vi "NUMPAD1_9(ПРОГРАММА).vi"(6 "МИНИМАЛЬНОЕ ЗНАЧЕНИЕ":dbl, 7 "МАКСИМАЛЬНОЕ ЗНАЧЕНИЕ":dbl, 8 "ДЛИННА СЛОВА":i8, 11 "ТЕКУЩЕЕ ЗНАЧЕНИЕ":string) -> (2 "НОВОЕ ЗНАЧЕНИЕ":string)   [LabVIEW 2016, in "Library.lvlib"]
uses:
  Granule-2000AT/PC/Library.lvlib
panel:
  in  ",":bool
  in  "ТЕМП":string
  in  "ОТМЕНА":bool
  in  "ВВОД":bool
  in  "УДАЛИТЬ":bool
  in  "0":bool
  in  "9":bool
  in  "8":bool
  in  "7":bool
  in  "6":bool
  in  "5":bool
  in  "4":bool
  in  "3":bool
  in  "2":bool
  in  "1":bool
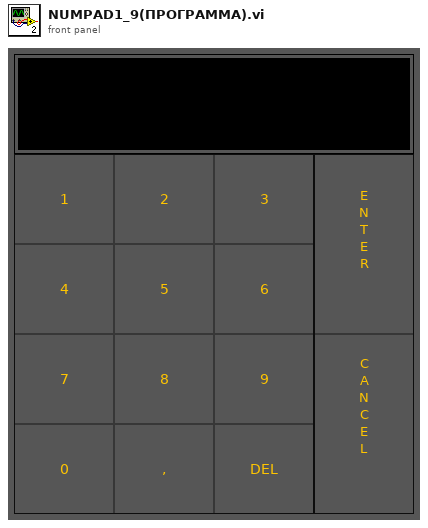
[diagram p1: front panel]
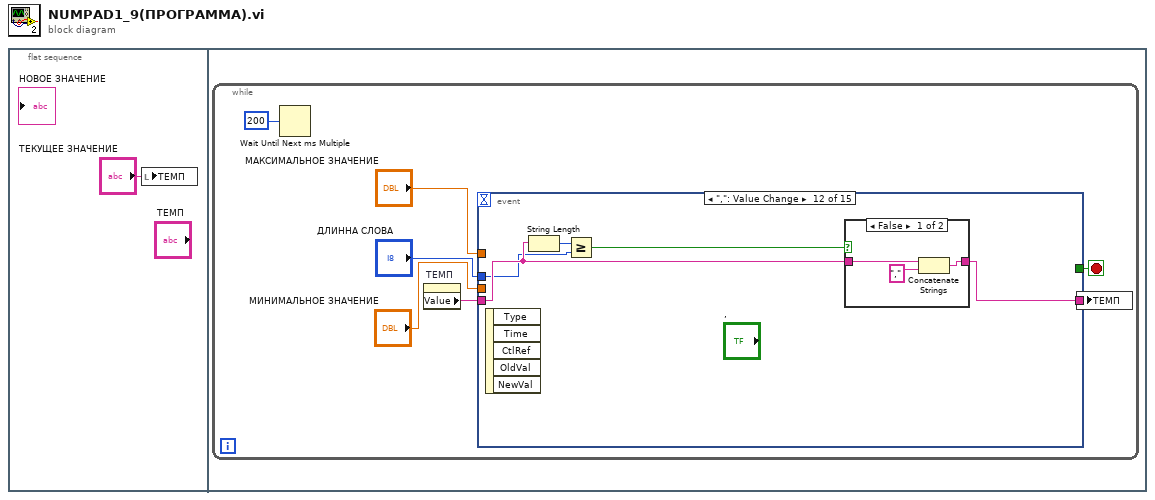
[diagram p0: block diagram]
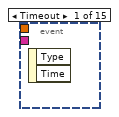
[diagram p2: hidden frame]
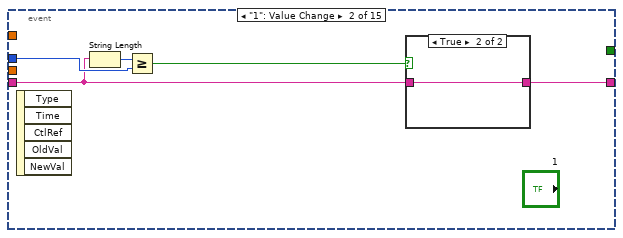
[diagram p3: hidden frame]
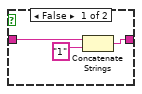
[diagram p4: hidden frame]
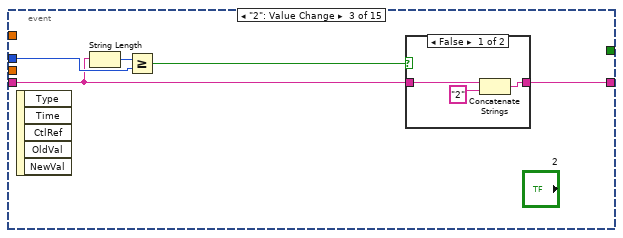
[diagram p5: hidden frame]
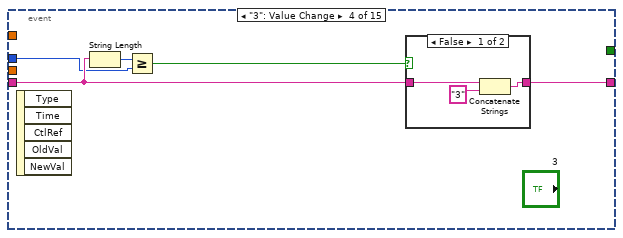
[diagram p7: hidden frame]
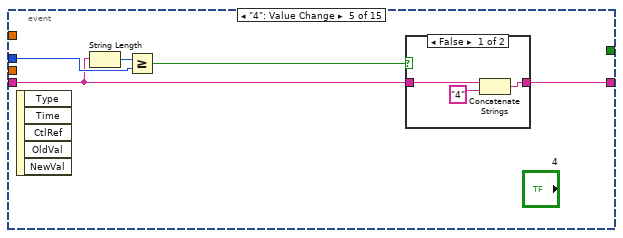
[diagram p9: hidden frame]
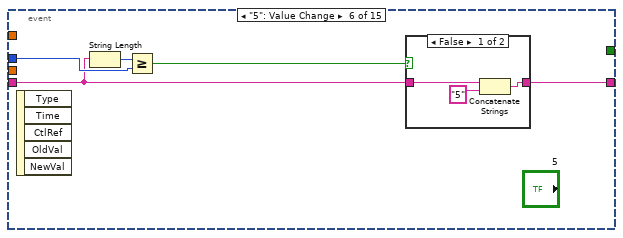
[diagram p11: hidden frame]
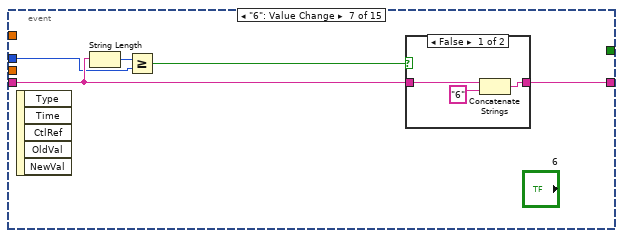
[diagram p13: hidden frame]
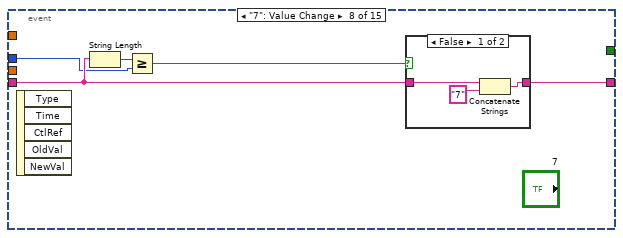
[diagram p15: hidden frame]
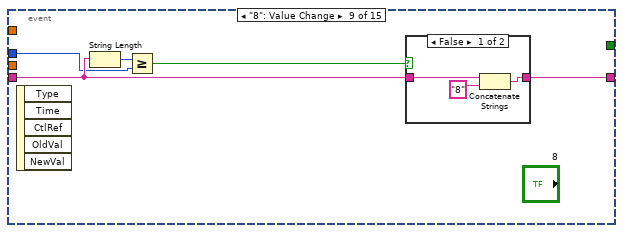
[diagram p17: hidden frame]
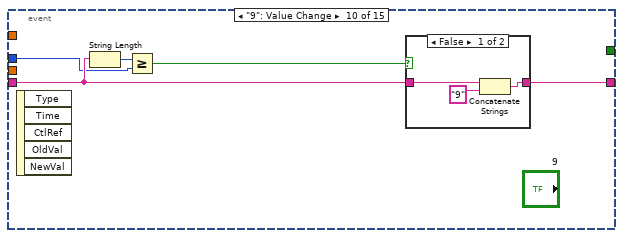
[diagram p19: hidden frame]
diagram:
  n1 = flat-sequence {
    frame #0 {
      n2 = local write "ТЕМП"("ТЕКУЩЕЕ ЗНАЧЕНИЕ") -> ()
    }
    frame #1 {
      n3 = while {
        stop <- w3 stop-if-true
        n4 = Wait Until Next ms Multiple(millisecond multiple=u32 200) -> ()  [unwired: 1 out]
        n5 = property on="ТЕМП" class="Str"() -> ("Value"=w7:string)  [unwired: 2 in, 2 out]
        n6 = event shown="[11] \",\": Value Change" {
          selector: _ -> [_ _ _ _ _ _ _ _ _ _ _ _ _ _ _]
          dyn-events: _ -> [_ _ _ _ _ _ _ _ _ _ _ _ _ _ _]
          timeout: _ -> [_ _ _ _ _ _ _ _ _ _ _ _ _ _ _]
          tunnel: "ДЛИННА СЛОВА" -> [_ w12 w20 w28 w38 w47 w55 w64 w72 w81 w91 w100 _ _ _]
          tunnel: w7 -> [_ w10 w19 w29 w37 w45 w56 w65 w74 w83 w92 w101 w109 w114 _]
          tunnel: [_ w9 w18 w27 w36 w46 w54 w63 w73 w82 w90 w99 w108 w112 _] -> w6
          tunnel: "МАКСИМАЛЬНОЕ ЗНАЧЕНИЕ" -> [_ _ _ _ _ _ _ _ _ _ _ _ _ w117 _]
          tunnel: "МИНИМАЛЬНОЕ ЗНАЧЕНИЕ" -> [_ _ _ _ _ _ _ _ _ _ _ _ _ w116 _]
          tunnel: [_ _ _ _ _ _ _ _ _ _ _ _ _ w113 "ОТМЕНА"] -> w3
          event Timeout {
            n7 = event-data() -> ()  [unwired: 1 in, 2 out]
          }
          event "1": Value Change {
            n8 = event-data() -> ()  [unwired: 1 in, 5 out]
            n9 = String Length(string=w10) -> (length=w13:i32)
            n10 = Greater Or Equal?(x=w13, y=w12) -> (x >= y?=w11:bool)
            n11 = case shown="True" w11 {
              tunnel: w10 -> [w16 w17]
              tunnel: [w14 w17] -> w9
              frame False {
                n12 = Concatenate Strings(w16, "1" ("string")) -> (w14:string)
              }
              frame True {
              }
            }
          }
          event "2": Value Change {
            n13 = event-data() -> ()  [unwired: 1 in, 5 out]
            n14 = String Length(string=w19) -> (length=w22:i32)
            n15 = Greater Or Equal?(x=w22, y=w20) -> (x >= y?=w21:bool)
            n16 = case shown="False" w21 {
              tunnel: w19 -> [w25 w26]
              tunnel: [w23 w26] -> w18
              frame False {
                n17 = Concatenate Strings(w25, "2" ("string")) -> (w23:string)
              }
              frame True {
              }
            }
          }
          event "3": Value Change {
            n18 = event-data() -> ()  [unwired: 1 in, 5 out]
            n19 = String Length(string=w29) -> (length=w31:i32)
            n20 = Greater Or Equal?(x=w31, y=w28) -> (x >= y?=w30:bool)
            n21 = case shown="False" w30 {
              tunnel: w29 -> [w34 w35]
              tunnel: [w32 w35] -> w27
              frame False {
                n22 = Concatenate Strings(w34, "3" ("string")) -> (w32:string)
              }
              frame True {
              }
            }
          }
          event "4": Value Change {
            n23 = event-data() -> ()  [unwired: 1 in, 5 out]
            n24 = String Length(string=w37) -> (length=w40:i32)
            n25 = Greater Or Equal?(x=w40, y=w38) -> (x >= y?=w39:bool)
            n26 = case shown="False" w39 {
              tunnel: w37 -> [w43 w44]
              tunnel: [w41 w44] -> w36
              frame False {
                n27 = Concatenate Strings(w43, "4" ("string")) -> (w41:string)
              }
              frame True {
              }
            }
          }
          event "5": Value Change {
            n28 = event-data() -> ()  [unwired: 1 in, 5 out]
            n29 = String Length(string=w45) -> (length=w49:i32)
            n30 = Greater Or Equal?(x=w49, y=w47) -> (x >= y?=w48:bool)
            n31 = case shown="False" w48 {
              tunnel: w45 -> [w52 w53]
              tunnel: [w50 w53] -> w46
              frame False {
                n32 = Concatenate Strings(w52, "5" ("string")) -> (w50:string)
              }
              frame True {
              }
            }
          }
          event "6": Value Change {
            n33 = event-data() -> ()  [unwired: 1 in, 5 out]
            n34 = String Length(string=w56) -> (length=w58:i32)
            n35 = Greater Or Equal?(x=w58, y=w55) -> (x >= y?=w57:bool)
            n36 = case shown="False" w57 {
              tunnel: w56 -> [w61 w62]
              tunnel: [w59 w62] -> w54
              frame False {
                n37 = Concatenate Strings(w61, "6" ("string")) -> (w59:string)
              }
              frame True {
              }
            }
          }
          event "7": Value Change {
            n38 = event-data() -> ()  [unwired: 1 in, 5 out]
            n39 = String Length(string=w65) -> (length=w67:i32)
            n40 = Greater Or Equal?(x=w67, y=w64) -> (x >= y?=w66:bool)
            n41 = case shown="False" w66 {
              tunnel: w65 -> [w70 w71]
              tunnel: [w68 w71] -> w63
              frame False {
                n42 = Concatenate Strings(w70, "7" ("string")) -> (w68:string)
              }
              frame True {
              }
            }
          }
          event "8": Value Change {
            n43 = event-data() -> ()  [unwired: 1 in, 5 out]
            n44 = String Length(string=w74) -> (length=w76:i32)
            n45 = Greater Or Equal?(x=w76, y=w72) -> (x >= y?=w75:bool)
            n46 = case shown="False" w75 {
              tunnel: w74 -> [w79 w80]
              tunnel: [w77 w80] -> w73
              frame False {
                n47 = Concatenate Strings(w79, "8" ("string")) -> (w77:string)
              }
              frame True {
              }
            }
          }
          event "9": Value Change {
            n48 = event-data() -> ()  [unwired: 1 in, 5 out]
            n49 = String Length(string=w83) -> (length=w85:i32)
            n50 = Greater Or Equal?(x=w85, y=w81) -> (x >= y?=w84:bool)
            n51 = case shown="False" w84 {
              tunnel: w83 -> [w88 w89]
              tunnel: [w86 w89] -> w82
              frame False {
                n52 = Concatenate Strings(w88, "9" ("string")) -> (w86:string)
              }
              frame True {
              }
            }
          }
          event "0": Value Change {
            n53 = event-data() -> ()  [unwired: 1 in, 5 out]
            n54 = String Length(string=w92) -> (length=w94:i32)
            n55 = Greater Or Equal?(x=w94, y=w91) -> (x >= y?=w93:bool)
            n56 = case shown="False" w93 {
              tunnel: w92 -> [w97 w98]
              tunnel: [w95 w98] -> w90
              frame False {
                n57 = Concatenate Strings(w97, "0" ("string")) -> (w95:string)
              }
              frame True {
              }
            }
          }
          event ",": Value Change {
            n58 = event-data() -> ()  [unwired: 1 in, 5 out]
            n59 = String Length(string=w101) -> (length=w103:i32)
            n60 = Greater Or Equal?(x=w103, y=w100) -> (x >= y?=w102:bool)
            n61 = case shown="False" w102 {
              tunnel: w101 -> [w106 w107]
              tunnel: [w104 w107] -> w99
              frame False {
                n62 = Concatenate Strings(w106, "," ("string")) -> (w104:string)
              }
              frame True {
              }
            }
          }
          event "УДАЛИТЬ": Value Change {
            n63 = event-data() -> ()  [unwired: 1 in, 5 out]
            n64 = String Length(string=w109) -> (length=w111:i32)
            n65 = Decrement(x=w111) -> (x-1=w110:i32)
            n66 = String Subset(string=w109, length (rest)=w110) -> (substring=w108:string)  [unwired: 1 in]
          }
          event "ВВОД": Value Change {
            n67 = event-data() -> ()  [unwired: 1 in, 5 out]
            n68 = Fract/Exp String To Number(string=w114) -> (number=w118:dbl)  [unwired: 3 in, 1 out]
            n69 = Greater Or Equal?(x=w118, y=w117) -> (x >= y?=w120:bool)
            n70 = Less Or Equal?(x=w118, y=w116) -> (x <= y?=w119:bool)
            n71 = Or(x=w120, y=w119) -> (x .or. y?=w115:bool)
            n72 = case shown="True" w115 {
              tunnel: w114 -> [w121 w123]
              tunnel: [TRUE FALSE] -> w113
              tunnel: [w121 w123] -> w112
              frame False {
                n73 = local write "НОВОЕ ЗНАЧЕНИЕ"(w121) -> ()
              }
              frame True {
                n74 = call "ЗНАЧЕНИЕ НЕКОР.vi"() -> ()  [unwired: 1 in]
              }
            }
          }
          event "ОТМЕНА": Value Change {
            n75 = event-data() -> ()  [unwired: 1 in, 5 out]
            n76 = property on="ТЕКУЩЕЕ ЗНАЧЕНИЕ" class="Str"() -> ("Value"=w126:string)  [unwired: 2 in, 2 out]
            n77 = local write "НОВОЕ ЗНАЧЕНИЕ"(w126) -> ()
          }
        }
        n78 = local write "ТЕМП"(w6) -> ()
      }
    }
  }
